vi "AM_Diode_Char_Sweep.vi"(4 "error in":errorcluster, 5 "R / kOhm":dbl, 6 "Vdelta / V":dbl, 7 "Vlow / V":dbl, 8 "Vhigh / V":dbl, 9 "VISA resource name 2":refnum<visa-resource-name>) -> (0 "error out":errorcluster, 1 "Idata":dbl[](array[numeric]), 2 "Vdata":dbl[](array[numeric]), 3 "VISA resource name 3":refnum<visa-resource-name>)   [LabVIEW 2019]
doc: "Perform DC voltage sweep for a diode characterisation using Arduino Micro\n\nAssumes circuit connected to Ch. A with BJT current amplifier\n\nMeasurement:\nA0 = Vr-hi, A1 = Vr-lo, A2 = A1 = Vd-hi, A3 = Vd-lo = Gnd (Not strictly necessary)\n\nOutput:\nIdata = A0 - A1 / R, Vdata = A3\n\nR. Sheehan 25 - 11 - 2020"
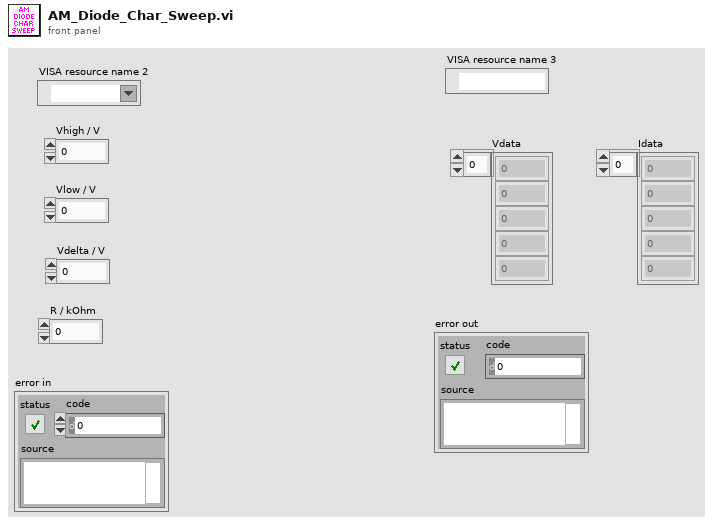
[diagram p1: front panel]
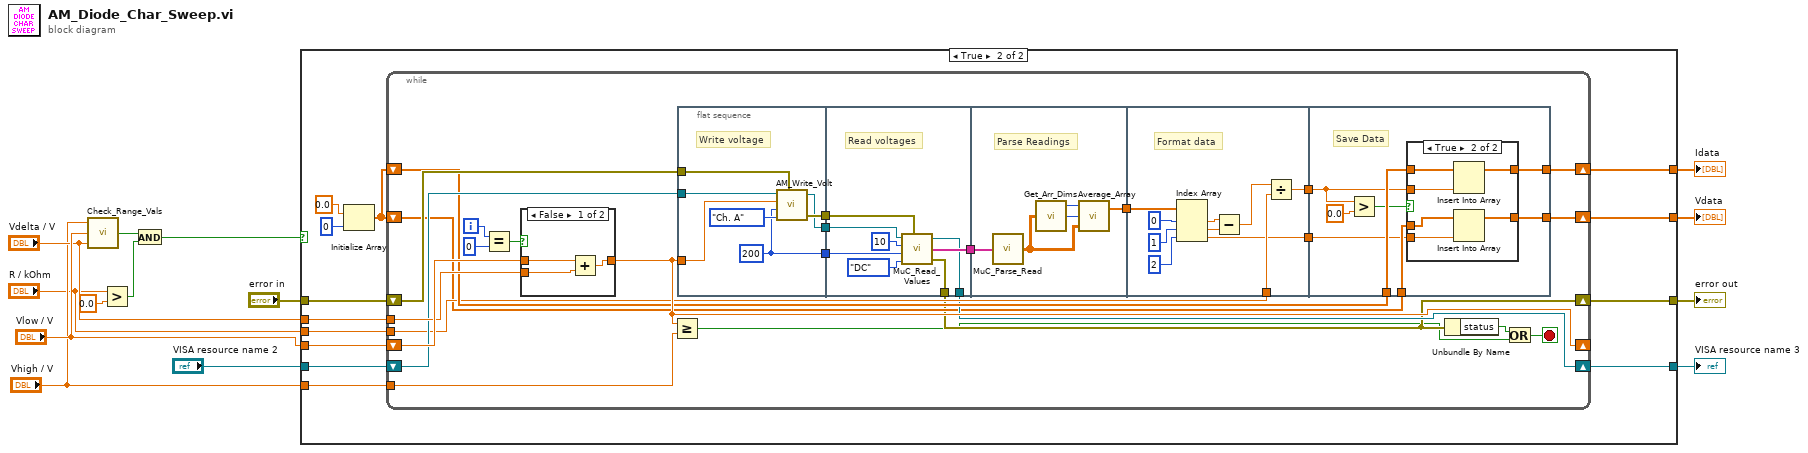
[diagram p0: block diagram]
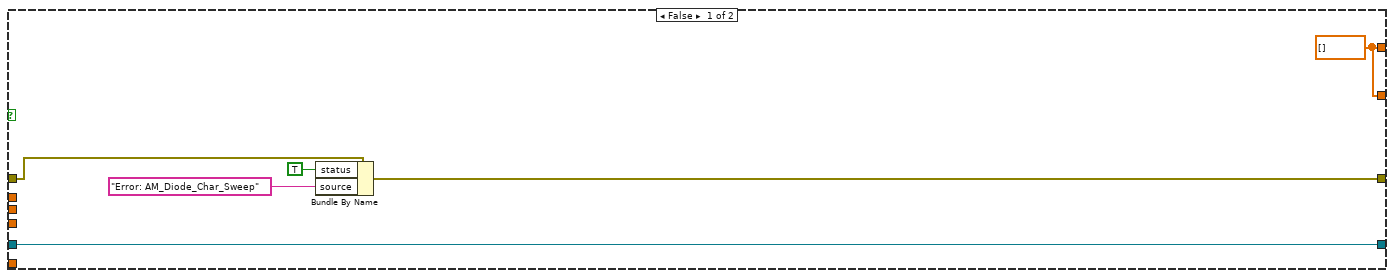
[diagram p2: hidden frame]
diagram:
  n1 = call "Check_Range_Vals.vi"("Increment"="Vdelta / V", "Lower Limit"="Vlow / V", "Upper Limit"="Vhigh / V") -> ("Bounds Are Good"=w3:bool)
  n2 = Greater?(x="R / kOhm", y=0.0) -> (0:w4:bool)
  n3 = And(x=w3, y=w4) -> (x .and. y?=w2:bool)
  n4 = case shown="True" w2 {
    tunnel: "Vlow / V" -> [_ w25]
    tunnel: "Vdelta / V" -> [_ w24]
    tunnel: "Vhigh / V" -> [_ w26]
    tunnel: "VISA resource name 2" -> [w20 w33]
    tunnel: "error in" -> [w18 w32]
    tunnel: [w20 w22] -> w9
    tunnel: [w17 w21] -> w8
    tunnel: [w19 w28] -> w7
    tunnel: [w19 w27] -> w6
    tunnel: "R / kOhm" -> [_ w23]
    frame False {
      w19 = dbl[] []
      n5 = Bundle By Name(cluster=w18, "status"=TRUE, "source"="Error: AM_Diode_Char_Sweep") -> (w17:errorcluster)
    }
    frame True {
      n6 = Initialize Array(0.0 ("element"), 0 ("dimension size")) -> (w29:dbl[])
      n7 = while {
        shift-right: [w49] -> _
        shift-left: w25 -> [w56]
        tunnel: w24 -> [w55]
        tunnel: w26 -> [w54]
        shift-right: [w47] -> w27
        shift-left: w29 -> [w48]
        shift-right: [w39] -> w28
        shift-left: w29 -> [w40]
        tunnel: w23 -> [w46]
        shift-right: [w41] -> w22
        shift-left: w33 -> [w51]
        shift-right: [w38] -> w21
        shift-left: w32 -> [w50]
        i -> [w58]
        stop <- w35 stop-if-true
        n8 = Equal?(x=w58, y=0) -> (x = y?=w59:bool)
        n9 = case shown="False" w59 {
          tunnel: w56 -> [w108 w109]
          tunnel: [w106 w109] -> w49
          tunnel: w55 -> [w107 _]
          frame False {
            n10 = Add(x=w108, y=w107) -> (x+y=w106:dbl)
          }
          frame True {
          }
        }
        n11 = Greater Or Equal?(x=w49, y=w54) -> (x >= y?=w36:bool)
        n12 = flat-sequence {
          tunnel: w51 -> [w66]
          tunnel: w50 -> [w65]
          tunnel: w49 -> [w64]
          tunnel: [w63] -> w43
          tunnel: [w62] -> w42
          tunnel: [w60] -> w34
          tunnel: [w74] -> w53
          tunnel: w43 -> [w71]
          tunnel: w42 -> [w70]
          tunnel: [w69] -> w41
          tunnel: [w68] -> w38
          tunnel: w34 -> [w67]
          tunnel: w53 -> [w75]
          tunnel: [w76] -> w52
          tunnel: w52 -> [w89]
          tunnel: w46 -> [w83]
          tunnel: [w82] -> w45
          tunnel: [w80] -> w44
          tunnel: w48 -> [w97]
          tunnel: w45 -> [w90]
          tunnel: w44 -> [w93]
          tunnel: w40 -> [w95]
          tunnel: [w94] -> w39
          tunnel: [w96] -> w47
          frame #0 {
            w60 = u32 200 ("Delay / ms")
            # "Write voltage"
            n13 = call "AM_Write_Volt.vi"("VISA resource name"=w66, "Volt / V"=w64, "Delay / ms"=w60, "Enum"=enum16{"Ch. A", "Ch. B"}."Ch. A", "error in (no error)"=w65) -> ("VISA resource name 2"=w62:refnum<visa-resource-name>, "error out"=w63:errorcluster)  [unwired: 1 out]
          }
          frame #1 {
            # "Read voltages"
            n14 = call "MuC_Read_Values.vi"("VISA resource name"=w70, "Nreads"=10, "Delay (ms)"=w67, "Read Type"=enum16{"DC", "AC"}."DC", "error in (no error)"=w71) -> ("VISA resource name 2"=w69:refnum<visa-resource-name>, "Buffer Data"=w74:string[], "error out"=w68:errorcluster)
          }
          frame #2 {
            # "Parse Readings"
            n15 = call "MuC_Parse_Read.vi"("Buffer Data"=w75) -> ("Data"=w79:dbl[][])
            n16 = call "Get_Arr_Dims.vi"("Data"=w79) -> ("N Rows"=w78:i32, "N Cols"=w77:i32)  [unwired: 1 out]
            n17 = call "Average_Array.vi"("Array"=w79, "Ncolumns"=w77, "Nrows"=w78) -> ("Average"=w76:dbl[])  [unwired: 1 out]
          }
          frame #3 {
            # "Format data"
            n18 = Index Array(array=w89, index #1=0 ("index"), index #2=1 ("index"), index #3=2 ("index")) -> (element #1=w86:dbl, element #2=w85:dbl, element #3=w80:dbl)
            n19 = Subtract(x=w86, y=w85) -> (x-y=w84:dbl)
            n20 = Divide(x=w84, y=w83) -> (x/y=w82:dbl)
          }
          frame #4 {
            # "Save Data"
            n21 = Greater?(x=w90, y=0.0) -> (0:w91:bool)
            n22 = case shown="True" w91 {
              tunnel: w97 -> [w99 w105]
              tunnel: [w99 w104] -> w96
              tunnel: w95 -> [w98 w103]
              tunnel: [w98 w102] -> w94
              tunnel: w93 -> [_ w101]
              tunnel: w90 -> [_ w100]
              frame False {
              }
              frame True {
                n23 = Insert Into Array(array=w105, new element=w100) -> (w104:dbl[])  [unwired: 1 in]
                n24 = Insert Into Array(array=w103, new element=w101) -> (w102:dbl[])  [unwired: 1 in]
              }
            }
          }
        }
        n25 = Unbundle By Name(w38) -> ("status"=w37:bool)
        n26 = Or(x=w37, y=w36) -> (x .or. y?=w35:bool)
      }
    }
  }
  "VISA resource name 3" <- w9
  "error out" <- w8
  "Vdata" <- w7
  "Idata" <- w6
